vi "AB_Engine_Update_Path.vi"(0 "old path":path, 5 "old paths":path[](array[path]), 7 "new paths":path[](array[path]), 9 "old dir paths":path[](array[path]), 11 "new dir paths":path[](array[path])) -> (4 "new path":path)   [LabVIEW 2020]
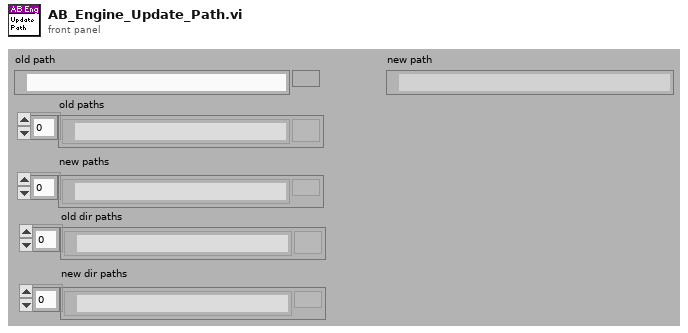
[diagram p1: front panel]
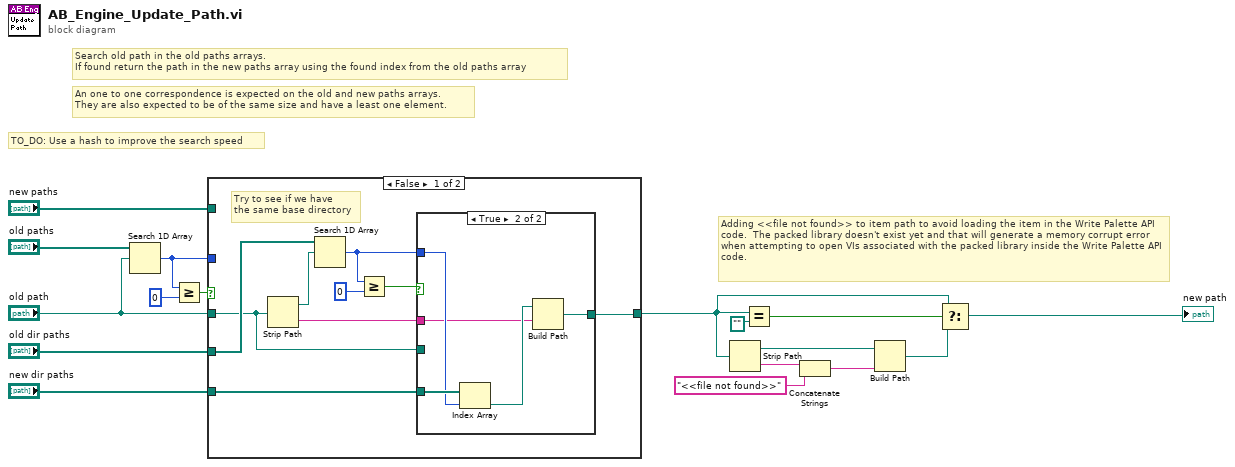
[diagram p0: block diagram]
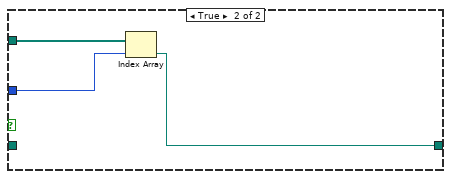
[diagram p3: hidden frame]
diagram:
  # "Adding <<file not found>> to item path to avoid loading the item in the Write Palette API code.  The packed library doesn't exist yet and that will generate a memory corrupt error when attempting to open VIs associated with the packed library inside the Write Palette API code."
  # "TO_DO: Use a hash to improve the search speed"
  # "An one to one correspondence is expected on the old and new paths arrays.\nThey are also expected to be of the same size and have a least one element."
  # "Search old path in the old paths arrays.\nIf found return the path in the new paths array using the found index from the old paths array"
  n1 = Search 1D Array(1D array="old paths", element="old path") -> (index of element=w12:i32)  [unwired: 1 in]
  n2 = Greater Or Equal?(x=w12, y=0) -> (x >= y?=w15:bool)
  n3 = case shown="False" w15 {
    tunnel: "new paths" -> [_ w35]
    tunnel: "old path" -> [w19 _]
    tunnel: w12 -> [_ w34]
    tunnel: [w18 w33] -> w4
    tunnel: "old dir paths" -> [w21 _]
    tunnel: "new dir paths" -> [w20 _]
    frame False {
      # "Try to see if we have \nthe same base directory"
      n4 = Strip Path(path=w19) -> (stripped path=w25:path, name=w23:string)
      n5 = Search 1D Array(1D array=w21, element=w25) -> (index of element=w22:i32)  [unwired: 1 in]
      n6 = Greater Or Equal?(x=w22, y=0) -> (x >= y?=w24:bool)
      n7 = case shown="True" w24 {
        tunnel: w23 -> [_ w29]
        tunnel: w22 -> [_ w31]
        tunnel: w20 -> [_ w32]
        tunnel: [w27 w28] -> w18
        tunnel: w19 -> [w27 _]
        frame False {
        }
        frame True {
          n8 = Index Array(array=w32, index=w31) -> (element=w30:path)
          n9 = Build Path(base path=w30, name or relative path=w29) -> (appended path=w28:path)
        }
      }
    }
    frame True {
      n10 = Index Array(array=w35, index=w34) -> (element=w33:path)
    }
  }
  n11 = Strip Path(path=w4) -> (stripped path=w5:path, name=w8:string)
  n12 = Equal?(x=w4, y=path "") -> (x = y?=w10:bool)
  n13 = Concatenate Strings(w8, "<<file not found>>" ("search string")) -> (w6:string)
  n14 = Build Path(base path=w5, name or relative path=w6) -> (appended path=w9:path)
  n15 = Select(t=w4, s=w10, f=w9) -> (s? t:f=→"new path":path)
